vi "Create queue.vi"(8 "error in":errorcluster, 11 "Comm Queue Name":string) -> (0 "error out":errorcluster, 3 "queue out":refnum<queue>)   [LabVIEW 2025, in "Queue API.lvlib"]
uses:
  Queue API.lvlib
  Controls/CAN Sending Data.ctl
  Controls/CAN Payload.ctl
  Commands.ctl
  Notifier Data.ctl
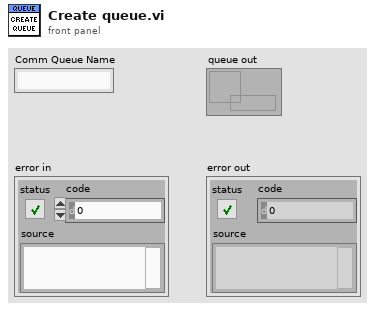
[diagram p1: front panel]
types:
  T1 = typedef "CAN Sending Data.ctl" = cluster{"Channel reference":u16, "MessagesToSend":cluster{"ID":u32, "MSGTYPE":u8, "LEN":u8, "DATA[0]":u8, "DATA[1]":u8, "DATA[2]":u8, "DATA[3]":u8, "DATA[4]":u8, "DATA[5]":u8, "DATA[6]":u8, "DATA[7]":u8}, "NoMessages":i32[], "Nexteer/XCP?":bool, "CAN Payload Array":T2[], "Expected responses":cluster{"DATA[0]":u8, "DATA[1]":u8, "DATA[2]":u8, "DATA[3]":u8}[], "Command":T3, "DATA[X]":u8[], "notifier out":refnum<notifier>}
  T2 = typedef "CAN Payload.ctl" = cluster{"DATA[0]":u8, "DATA[1]":u8, "DATA[2]":u8, "DATA[3]":u8, "DATA[4]":u8, "DATA[5]":u8, "DATA[6]":u8, "DATA[7]":u8}
  T3 = typedef "Commands.ctl" = enum16{"Nexteer connect", "Write Polarity", "Write BEMF", "Write Torque Scale Sensors T1", "Write Torque Scale Sensors T2", "Trim HW Torque Sensors T1", "Trim HW Torque Sensors T2", "Read HW Torque Trim Performed Sensors T1", "Read HW Torque Trim Performed Sensors T2", "Write EOL Offset values to defaults", "Write EOL Gain values to defaults", "Write Serial Number", "Write Hardware Part Number", "Write EPS Serial Number", "Read MEC Counter", "MCU Reset", "Read System State", "Read First Motor Position", "Manufacturing Diagnostic Defeat", "Perform Current Offset ", "Current Offset Status", "Enable Engine Run", "Perform Current Gain ", "Current Gain Status", "Disable Torque Ramp Down ", "Disable Engine Run", "Set Vehicle Speed Override", "Read Offset Values Using FD F5", "Read Gain Values Using FD F4", "Clear Nexteer NTCs", "Read Second Motor Position", "Read ECU Software ID", "Read Internal Software Version", "Read Bootloader ID", "Read Bootloader Software Version", "Read Calibration Release 0", "Read Calibration Release 1", "Read Calibration Release 2", "Read Temperature  ", "Battery Voltage  ", "Read Motor Angle 0", "Read Motor Angle 1 ", "Set Motor Torque Command ", "Read Motor Current   ", "Stop Motor Torque Command", "Read NTCs", "Read Serial Number", "Read HW Part Number", "Read Polarity", "Set NVM Access Defeat", "Read Software Release", "Read Software Build Date", "Write Single Inverter Hardware value", "Write Dual Inverter Hardware value", "Read Single Inverter HW Value", "Read Dual Inverter HW Value", "Write MEC Counter FE", "Write MEC Counter FF", "Read BEMF", "Read Torque 1 FDB6", "Read Torque 2 FDB7", "Read Torque Trim 1 FDB4", "Read Torque Trim 2 FDB5", "Write Torque Trim 1 FDB4", "Write Torque Trim 2 FDB5", "XCP connect", "Read HW Torque T1", "Read HW Torque T2", "Read Motor Speed "}
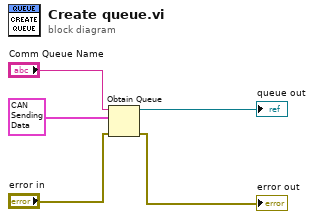
[diagram p0: block diagram]
diagram:
  n1 = Obtain Queue(name (unnamed)="Comm Queue Name", element data type=T1 {"Channel reference"=0, "MessagesToSend"={"ID"=0, "MSGTYPE"=0, "LEN"=0, "DATA[0]"=0, "DATA[1]"=0, "DATA[2]"=0, "DATA[3]"=0, "DATA[4]"=0, "DATA[5]"=0, "DATA[6]"=0, "DATA[7]"=0}, "NoMessages"=[], "Nexteer/XCP?"=FALSE, "CAN Payload Array"=[], "Expected responses"=[], "Command"=enum."MCU Reset", "DATA[X]"=[], "notifier out"=refnum}, error in (no error)="error in") -> (queue out=→"queue out":refnum<queue>, error out=→"error out":errorcluster)  [unwired: 2 in, 1 out]
